vi "Create.vi"(8 "error in (no error)":errorcluster, 10 "PlayerFolder":path, 11 "PlayerName":string) -> (0 "error out":errorcluster, 3 "Player out":refnum<class "Player.lvclass">)   [LabVIEW 2015, in "TronviewGame.lvlib" / "Player.lvclass"]
uses:
  Player.lvclass
  Player.lvclass/Player.ctl
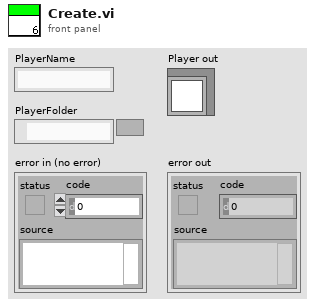
[diagram p1: front panel]
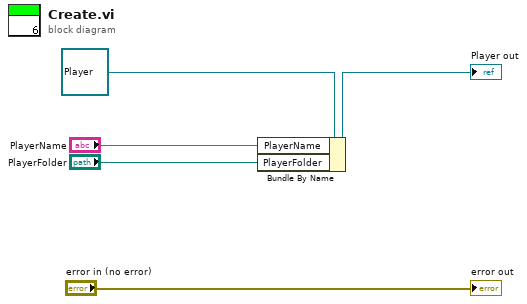
[diagram p0: block diagram]
diagram:
  n1 = Bundle By Name(cluster=refnum<class "Player.lvclass"> refnum ("Player in"), "PlayerName"="PlayerName", "PlayerFolder"="PlayerFolder") -> (→"Player out":refnum<class "Player.lvclass">)
  "error out" <- "error in (no error)"
